vi "Const o keyword.vi"() -> (3 "Const o keyword":string[](array[string]))   [LabVIEW 2018, in "Data Parser.lvclass"]
uses:
  Data Parser.lvclass
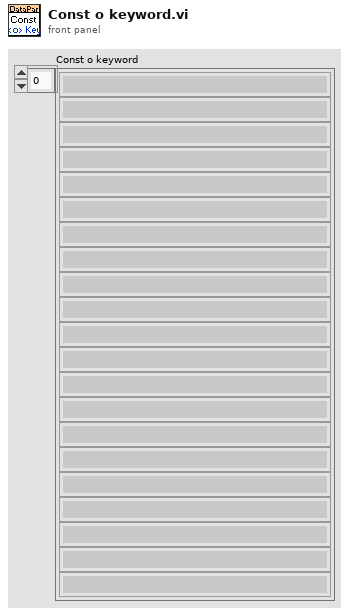
[diagram p1: front panel]
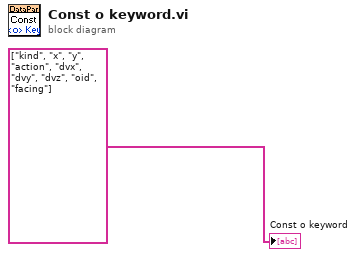
[diagram p0: block diagram]
diagram:
  "Const o keyword" <- string[] ["kind", "x", "y", "action", "dvx", "dvy", "dvz", "oid", "facing"]
